vi "Lake Shore 331 Temperature Controller.vi"(1 "Loop (0: 1)":u16(ring) items=["1", "2"], 2 "Gain (P)":dbl=50.0 min=0.0 max=1000.0 step=0.1 format="%.1f", 3 "Reset (I)":dbl=50.0 min=0.0 max=1000.0 step=0.1 format="%.1f", 4 "Rate (D)":dbl=100.0 min=0.0 max=200.0 step=1.0, 7 "Manual Output":dbl min=0.0 max=100.0 step=0.001 format="%.3f", 9 "Heater Range (0: Off)":u16(ring) items=["Off", "Low (0.5W)", "Med (5W)", "High (50W)"]) -> (16 "Sensor A":dbl=308.03 min=0.0 max=1645.0 step=1e-05 format="%.5f", 18 "Heater Output":dbl(slide) min=0.0 max=100.0 step=0.01 scale=0.0..100.0 scale format="%.1f")   [LabVIEW 2015]
doc: "This VI was designed to demonstrate typical usage of sub vi's containing the more common 331 functions.\n\nThis example configures the loop and setpoint of the instrument, allows for a delay, and then reads sensor and heater output data. The user is given the option of just reading data and not configuring the instrument."
uses:
  <instrlib>/Lake Shore Cryotronics 331/Lake Shore Cryotronics 331.lvlib
panel:
  out "In Range":bool=TRUE
  in  "Wait Time":dbl=30.0 min=0.0 max=1000.0 step=0.1 format="%.1f"
  in  "Tolerance":dbl=0.1 min=0.0 max=1000.0 step=0.1 format="%.1f"
  in  "Setpoint":dbl=308.0 min=-273.0 max=300000.0 step=0.0001 format="%.4f"
  in  "Control Mode (0: Manual PID)":u16(ring) items=["Manual PID", "Zone", "Open Loop", "AutoTune PID", "AutoTune PI", "AutoTune P"]
  in  "Input to \nControl From":u16(ring) items=["A", "B"]
  out "Loop 1 Heater Range":u16(ring) items=["Off", "Low (0.5W)", "Med (5W)", "High (50W)"]
  out "Manual Output":dbl min=0.0 max=100.0 step=0.001 format="%.3f"
  out "Rate (D)":dbl=100.0 min=0.0 max=1000.0 step=0.1 format="%.1f"
  out "Reset (I)":dbl=50.0 min=0.0 max=1000.0 step=0.1 format="%.1f"
  out "Gain (P)":dbl=50.0 min=0.0 max=1000.0 step=0.1 format="%.1f"
  out "Auto Tuning":bool
  in  "Set":bool
  in  "stop":bool
  out "Waveform Chart":T1(graph)={"Kelvin Reading"=307.41, "Kelvin Reading"=308.03, "Setpoint"=308.0}
  out "Sensor B":dbl=307.41 min=0.0 max=1645.0 step=1e-05 format="%.5f"
  in  "VISA resource name":refnum<visa-resource-name>="COM4"
  # "%"
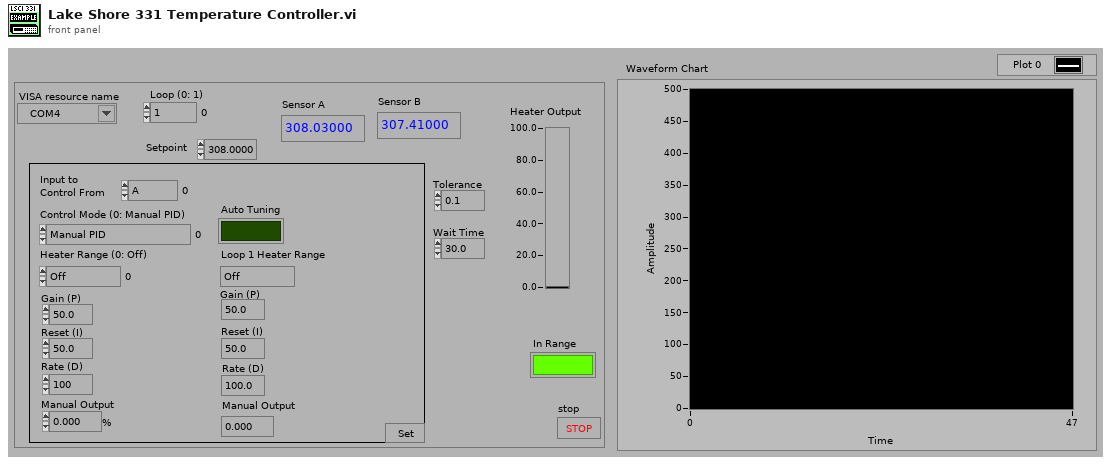
[diagram p1: front panel]
types:
  T1 = cluster{"Kelvin Reading":dbl, "Kelvin Reading":dbl, "Setpoint":dbl}
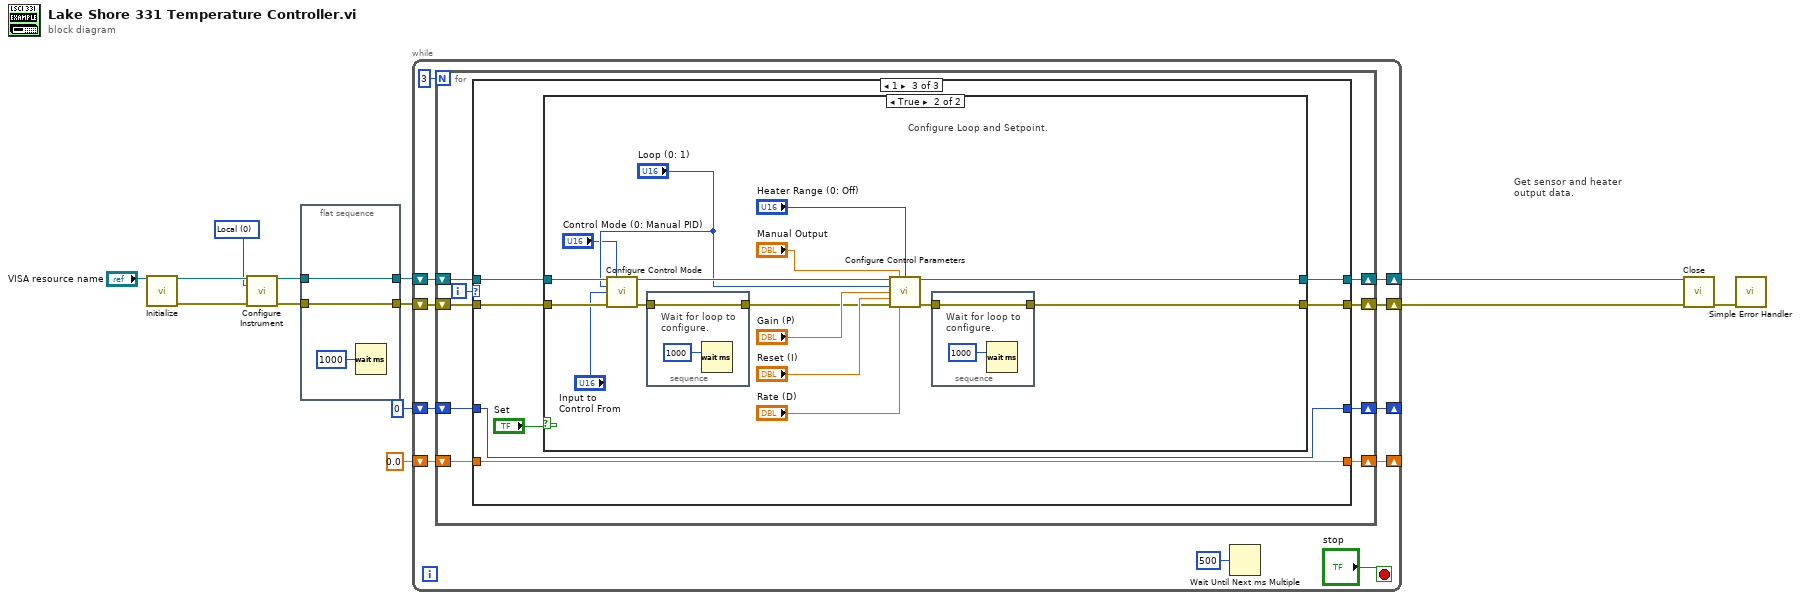
[diagram p0: block diagram]
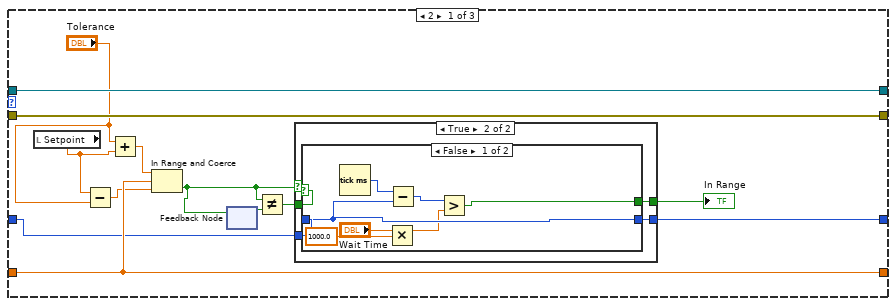
[diagram p2: hidden frame]
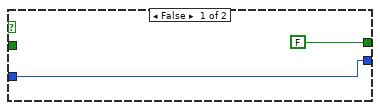
[diagram p3: hidden frame]
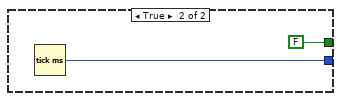
[diagram p4: hidden frame]
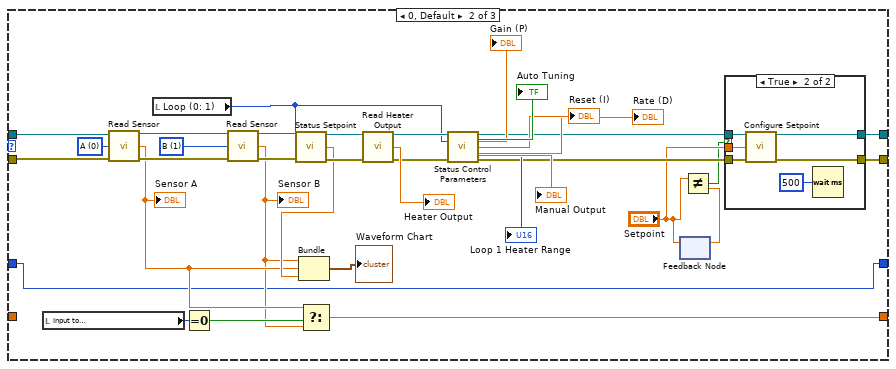
[diagram p5: hidden frame]
diagram:
  w7 = u16 0 items=["Local", "Remote", "Remote w/ Lockout"] ("Remote Interface\nMode (0: Local)")
  # "Get sensor and heater\noutput data."
  n1 = call <instrlib>:"Initialize.vi"("VISA resource name"="VISA resource name") -> ("VISA resource name out"=w9:refnum<visa-resource-name>, "error out"=w8:errorcluster)  [unwired: 13 in]
  n2 = call <instrlib>:"Configure Instrument.vi"("VISA resource name"=w9, "Remote Interface\nMode (0: Local)"=w7, "error in (no error)"=w8) -> ("VISA resource name out"=w6:refnum<visa-resource-name>, "error out"=w4:errorcluster)  [unwired: 11 in]
  n3 = flat-sequence {
    tunnel: w6 -> [w16]
    tunnel: [w16] -> w5
    tunnel: w4 -> [w15]
    tunnel: [w15] -> w3
    frame #0 {
      n4 = Wait (ms)(milliseconds to wait=u32 1000) -> ()  [unwired: 1 out]
    }
  }
  n5 = while {
    shift-right: [w25] -> w11
    shift-left: w5 -> [w27]
    shift-right: [w24] -> w10
    shift-left: w3 -> [w26]
    shift-right: [w20] -> _
    shift-left: 0.0 ("Kelvin Reading") -> [w19]
    shift-right: [w18] -> _
    shift-left: u32 0 ("millisecond timer value") -> [w17]
    stop <- "stop" stop-if-true
    n6 = for {
      N: 3 -> [_]
      shift-right: [w34] -> w25
      shift-left: w27 -> [w36]
      shift-right: [w33] -> w24
      shift-left: w26 -> [w35]
      shift-right: [w31] -> w20
      shift-left: w19 -> [w30]
      shift-right: [w29] -> w18
      shift-left: w17 -> [w28]
      i -> [w32]
      n7 = case shown="1" w32 {
        tunnel: w36 -> [w49 w99 w114]
        tunnel: w35 -> [w48 w98 w113]
        tunnel: [w49 w74 w112] -> w34
        tunnel: [w48 w75 w111] -> w33
        tunnel: [w47 w66 w109] -> w31
        tunnel: w30 -> [w47 _ w109]
        tunnel: [w38 w65 w108] -> w29
        tunnel: w28 -> [w37 w65 w108]
        frame 2 {
          n8 = local read "Setpoint"() -> (w45:dbl)
          n9 = Subtract(x=w45, y="Tolerance") -> (x-y=w43:dbl)
          n10 = Add(x="Tolerance", y=w45) -> (x+y=w46:dbl)
          n11 = In Range and Coerce(upper limit=w46, x=w47, lower limit=w43) -> (In Range?=w41:bool)  [unwired: 1 out]
          n12 = feedback #1() -> (w40:bool)  [unwired: 1 in]
          n13 = feedback-in #1(w41) -> ()
          n14 = Not Equal?(x=w41, y=w40) -> (x != y?=w39:bool)
          n15 = case shown="True" w41 {
            tunnel: [FALSE ("In Range") w52] -> w42
            tunnel: w39 -> [_ w55]
            tunnel: [w50 w54] -> w38
            tunnel: w37 -> [w50 w53]
            frame False {
            }
            frame True {
              n16 = case shown="False" w55 {
                tunnel: [w58 w64] -> w54
                tunnel: w53 -> [w58 _]
                tunnel: [w59 FALSE ("In Range")] -> w52
                frame False {
                  n17 = Tick Count (ms)() -> (millisecond timer value=w62:u32)
                  n18 = Multiply(x="Wait Time", y=1000.0) -> (x*y=w57:dbl)
                  n19 = Subtract(x=w62, y=w58) -> (x-y=w61:u32)
                  n20 = Greater?(x=w61, y=w57) -> (0:w59:bool)
                }
                frame True {
                  n21 = Tick Count (ms)() -> (millisecond timer value=w64:u32)
                }
              }
            }
          }
          "In Range" <- w42
        }
        frame 0, Default {
          w94 = u16 1 items=["A", "B"] ("Input (0: A)")
          w97 = u16 0 items=["A", "B"] ("Input (0: A)")
          n22 = local read "Input to \nControl From"() -> (w70:u16)
          n23 = call <instrlib>:"Read Sensor.vi"("VISA resource name"=w99, "Input (0: A)"=w97, "error in (no error)"=w98) -> ("VISA resource name out"=w96:refnum<visa-resource-name>, "Kelvin Reading"=w68:dbl, "error out"=w95:errorcluster)  [unwired: 8 in, 2 out]
          "Sensor A" <- w68
          n24 = local read "Loop (0: 1)"() -> (w78:u16)
          n25 = Equal To 0?(x=w70) -> (x = 0?=w69:bool)
          n26 = call <instrlib>:"Read Sensor.vi"("VISA resource name"=w96, "Input (0: A)"=w94, "error in (no error)"=w95) -> ("VISA resource name out"=w91:refnum<visa-resource-name>, "Kelvin Reading"=w67:dbl, "error out"=w89:errorcluster)  [unwired: 8 in, 2 out]
          "Sensor B" <- w67
          n27 = call <instrlib>:"Status Setpoint.vi"("VISA resource name"=w91, "Loop (0: 1)"=w78, "error in (no error)"=w89) -> ("VISA resource name out"=w90:refnum<visa-resource-name>, "Setpoint"=w87:dbl, "error out"=w88:errorcluster)  [unwired: 10 in]
          n28 = Bundle("Kelvin Reading"=w67, "Kelvin Reading"=w68, "Setpoint"=w87) -> (→"Waveform Chart":T1)  [unwired: 1 in]
          n29 = Select(t=w68, s=w69, f=w67) -> (s? t:f=w66:dbl)
          n30 = call <instrlib>:"Read Heater Output.vi"("VISA resource name"=w90, "error in (no error)"=w88) -> ("VISA resource name out"=w86:refnum<visa-resource-name>, "Loop 1\nHeater Output"=→"Heater Output":dbl, "error out"=w85:errorcluster)  [unwired: 11 in]
          n31 = call <instrlib>:"Status Control Parameters.vi"("VISA resource name"=w86, "Loop (0: 1)"=w78, "error in (no error)"=w85) -> ("Loop 1 Tuning Status"=→"Auto Tuning":bool, "VISA resource name out"=w77:refnum<visa-resource-name>, "Gain (P)"=→"Gain (P)":dbl, "Reset (I)"=→"Reset (I)":dbl, "Rate (D)"=→"Rate (D)":dbl, "Loop 1 Heater Range"=→"Loop 1 Heater Range":u16, "Manual Output (0.000 %)"=→"Manual Output":dbl, "error out"=w76:errorcluster)  [unwired: 5 in]
          n32 = feedback-in #2("Setpoint") -> ()
          n33 = feedback #2() -> (w72:dbl)  [unwired: 1 in]
          n34 = Not Equal?(x="Setpoint", y=w72) -> (x != y?=w71:bool)
          n35 = case shown="True" w71 {
            tunnel: w77 -> [w100 w107]
            tunnel: w76 -> [w101 w106]
            tunnel: [w101 w105] -> w75
            tunnel: [w100 w104] -> w74
            tunnel: "Setpoint" -> [_ w103]
            frame False {
            }
            frame True {
              n36 = call <instrlib>:"Configure Setpoint.vi"("VISA resource name"=w107, "Setpoint (0.0000)"=w103, "error in (no error)"=w106) -> ("VISA resource name out"=w104:refnum<visa-resource-name>, "error out"=w105:errorcluster)  [unwired: 11 in]
              n37 = Wait (ms)(milliseconds to wait=u32 500) -> ()  [unwired: 1 out]
            }
          }
        }
        frame 1 {
          n38 = case shown="True" "Set" {
            tunnel: w113 -> [w115 w124]
            tunnel: w114 -> [w116 w126]
            tunnel: [w115 w119] -> w111
            tunnel: [w116 w120] -> w112
            frame False {
              # "Do not configure Loop and Setpoint."
            }
            frame True {
              # "Configure Loop and Setpoint."
              n39 = call <instrlib>:"Configure Control Mode.vi"("VISA resource name"=w126, "Control Mode (0: Manual PID)"="Control Mode (0: Manual PID)", "Loop (0: 1)"="Loop (0: 1)", "Input to \nControl From (0: A)"="Input to \nControl From", "error in (no error)"=w124) -> ("VISA resource name out"=w125:refnum<visa-resource-name>, "error out"=w118:errorcluster)  [unwired: 9 in]
              n40 = stacked-sequence {
                tunnel: w118 -> [w133]
                tunnel: [w133] -> w117
                frame #0 {
                  # "Wait for loop to \nconfigure."
                  n41 = Wait (ms)(milliseconds to wait=u32 1000) -> ()  [unwired: 1 out]
                }
              }
              n42 = call <instrlib>:"Configure Control Parameters.vi"("VISA resource name"=w125, "Manual Output (0.000 %)"="Manual Output", "Heater Range (0: Off)"="Heater Range (0: Off)", "Loop (0: 1)"="Loop (0: 1)", "Gain (P) (0.0)"="Gain (P)", "Reset (I) (0.0)"="Reset (I)", "error in (no error)"=w117, "Rate (D) (0)"="Rate (D)") -> ("VISA resource name out"=w120:refnum<visa-resource-name>, "error out"=w132:errorcluster)  [unwired: 6 in]
              n43 = stacked-sequence {
                tunnel: w132 -> [w135]
                tunnel: [w135] -> w119
                frame #0 {
                  # "Wait for loop to \nconfigure."
                  n44 = Wait (ms)(milliseconds to wait=u32 1000) -> ()  [unwired: 1 out]
                }
              }
            }
          }
        }
      }
    }
    n45 = Wait Until Next ms Multiple(millisecond multiple=u32 500) -> ()  [unwired: 1 out]
  }
  n46 = call <instrlib>:"Close.vi"("VISA resource name"=w11, "error in (no error)"=w10) -> ("error out"=w13:errorcluster)  [unwired: 13 in]
  n47 = call <vilib>:"Simple Error Handler.vi"("error in (no error)"=w13) -> ()  [unwired: 4 in, 5 out]
